vi "2 angle_difference.vi"(1 "Angle 2":dbl, 2 "Angle 1":dbl) -> (0 "Difference":dbl)   [LabVIEW 2011]
doc: "Returns the angle between to headings, accounting for wraparound (0 and 355 are 5 degrees apart)"
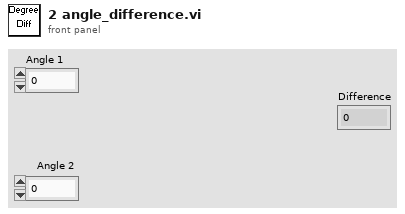
[diagram p1: front panel]
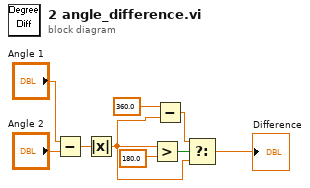
[diagram p0: block diagram]
diagram:
  n1 = Subtract(x="Angle 1", y="Angle 2") -> (x-y=w3:dbl)
  n2 = Absolute Value(x=w3) -> (abs(x)=w1:dbl)
  n3 = Greater?(x=w1, y=180.0) -> (0:w7:bool)
  n4 = Subtract(x=360.0 ("y"), y=w1) -> (x-y=w4:dbl)
  n5 = Select(t=w4, s=w7, f=w1) -> (s? t:f=→"Difference":dbl)
